vi "JoinPics.vi"(7 "Mode":enum16{"Horizontal", "Vertical"}(ring), 10 "Array-o-pix":picture[](array[picture])) -> (2 "JoinedPics":picture)   [LabVIEW 2021]
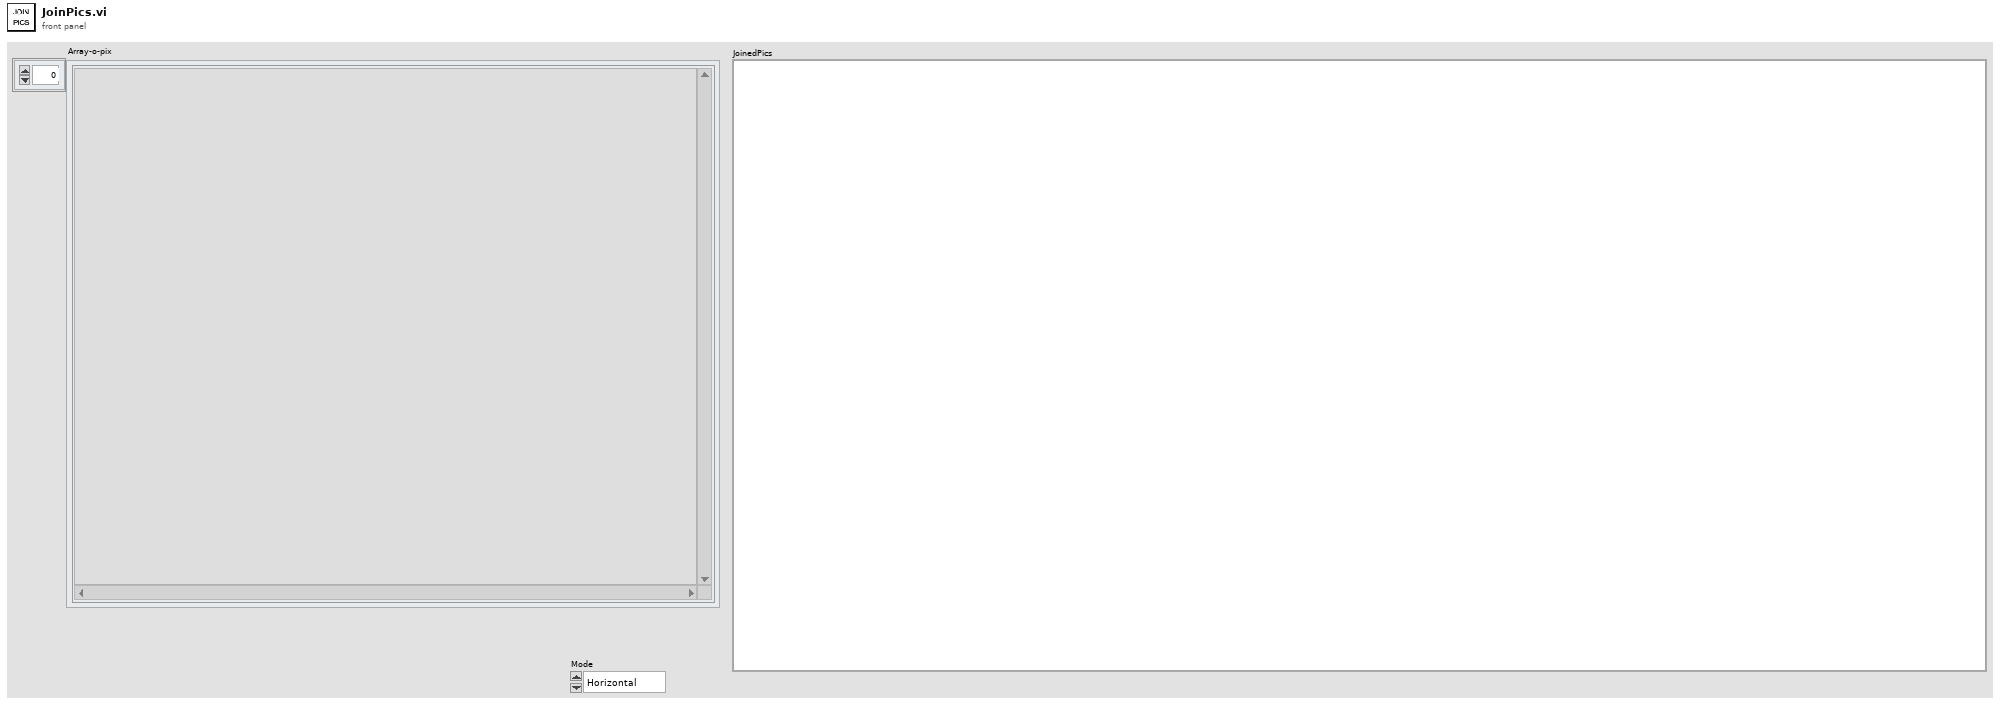
[diagram p1: front panel]
types:
  T1 = typedef "imagedata.ctl" = cluster{"image type":i32, "image depth":i32, "image":u8[], "mask":u8[], "colors":u32[], "Rectangle":cluster{"left":i16, "top":i16, "right":i16, "bottom":i16}}
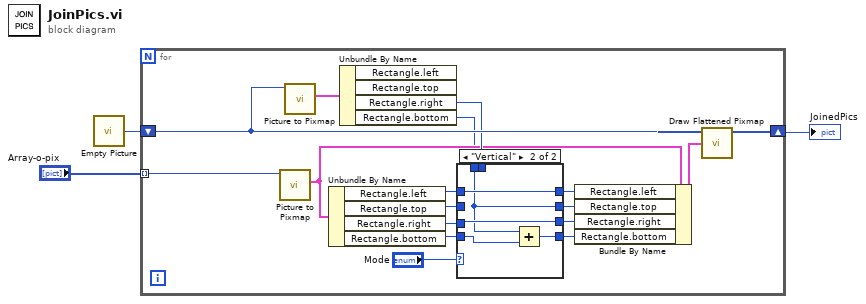
[diagram p0: block diagram]
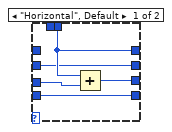
[diagram p2: hidden frame]
diagram:
  n1 = call "Empty Picture"() -> ("empty picture"=w2:picture)
  n2 = for {
    tunnel: "Array-o-pix" -> [w4] mode=indexing
    shift-right: [w20] -> w3
    shift-left: w2 -> [w19]
    n3 = call <vilib>:"Picture to Pixmap.vi"("picture"=w4) -> ("image data"=w14:T1)  [unwired: 9 in, 1 out]
    n4 = call <vilib>:"Picture to Pixmap.vi"("picture"=w19) -> ("image data"=w18:T1)  [unwired: 9 in, 1 out]
    n5 = Unbundle By Name(w14) -> ("Rectangle.left"=w5:i16, "Rectangle.top"=w10:i16, "Rectangle.right"=w15:i16, "Rectangle.bottom"=w8:i16)
    n6 = Unbundle By Name(w18) -> ("Rectangle.right"=w16:i16, "Rectangle.bottom"=w6:i16)  [unwired: 2 out]
    n7 = case shown="\"Vertical\"" "Mode" {
      tunnel: [w25 w29] -> w17
      tunnel: w16 -> [w23 _]
      tunnel: w15 -> [w24 w29]
      tunnel: [w23 w30] -> w11
      tunnel: w10 -> [w22 _]
      tunnel: [w22 w27] -> w9
      tunnel: w8 -> [w21 w26]
      tunnel: [w21 w28] -> w7
      tunnel: w6 -> [_ w27]
      tunnel: w5 -> [_ w30]
      frame "Horizontal", Default {
        n8 = Add(x=w23, y=w24) -> (x+y=w25:i16)
      }
      frame "Vertical" {
        n9 = Add(x=w27, y=w26) -> (x+y=w28:i16)
      }
    }
    n10 = Bundle By Name(cluster=w14, "Rectangle.left"=w11, "Rectangle.top"=w9, "Rectangle.right"=w17, "Rectangle.bottom"=w7) -> (w13:T1)
    n11 = call <vilib>:"Draw Flattened Pixmap.vi"("image data"=w13, "picture"=w19) -> ("new picture"=w20:picture)  [unwired: 7 in]
  }
  "JoinedPics" <- w3
